vi "csmdoc_import_all_csm_VI_description_doc.vi"() -> ()   [LabVIEW 2017, in "csmdoc.lvlib"]
uses:
  csmdoc.lvlib
  _Shared/CSM Shared.lvlib
panel:
  out "Numeric":i32=317
  in  "LANG ID":string="EN"
  in  "Error in":errorcluster caption="error in (no error)"
  out "error out":errorcluster
  out "Array":path[](array[path])
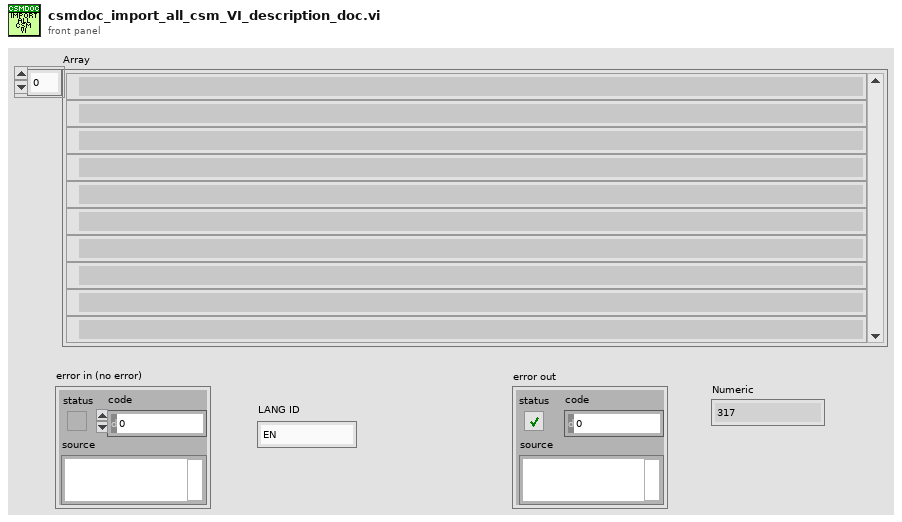
[diagram p1: front panel]
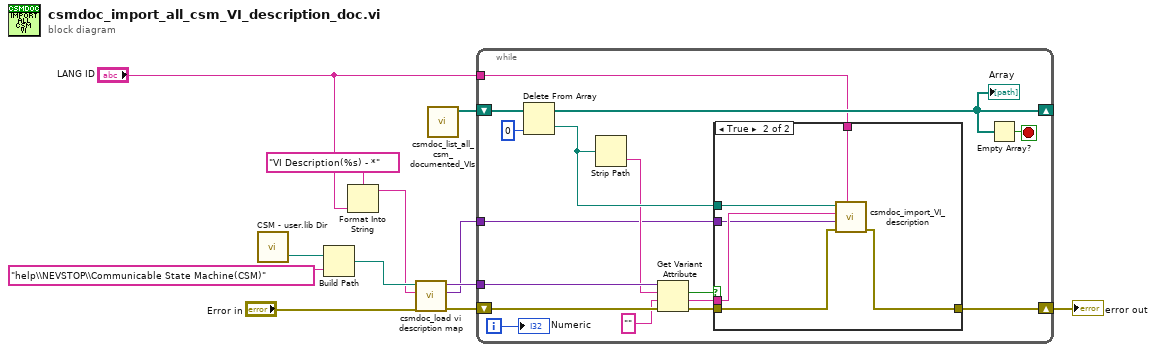
[diagram p0: block diagram]
diagram:
  n1 = call "CSM - user.lib Dir.vi"() -> ("<LabVIEW>"=w5:path)  [unwired: 2 in, 1 out]
  n2 = Build Path(base path=w5, name or relative path="help\\NEVSTOP\\Communicable State Machine(CSM)") -> (appended path=w4:path)
  n3 = Format Into String(format string="VI Description(%s) - *" ("pattern"), "LANG ID") -> (resulting string=w1:string)  [unwired: 2 in, 1 out]
  n4 = call "csmdoc_load vi description map.vi"("Error In"="Error in", "Pattern"=w1, "Path"=w4) -> ("error out"=w10:errorcluster, "NoteMap"=w7:variant, "DescMap"=w11:variant)  [unwired: 6 in]
  n5 = call "csmdoc_list_all_csm_documented_VIs.vi"() -> ("Array"=w12:path[])  [unwired: 11 in]
  n6 = while {
    shift-right: [w25] -> _
    shift-left: w12 -> [w27]
    tunnel: w11 -> [w23]
    shift-right: [w18] -> w9
    shift-left: w10 -> [w20]
    tunnel: w7 -> [w15]
    tunnel: "LANG ID" -> [w14]
    i -> [w13]
    stop <- w26 stop-if-true
    n7 = Delete From Array(array=w27, index=0) -> (deleted portion=w28:path, array with subset deleted=w25:path[])  [unwired: 1 in]
    "Array" <- w25
    n8 = Strip Path(path=w28) -> (name=w22:string)  [unwired: 1 out]
    n9 = Get Variant Attribute(Variant=w23, name=w22, default value (empty Variant)="" ("String"), error in=w20) -> (found=w21:bool, value=w16:string, error out=w19:errorcluster)  [unwired: 1 out]
    n10 = case shown="True" w21 {
      tunnel: w28 -> [_ w35]
      tunnel: w19 -> [w29 w34]
      tunnel: [w29 w33] -> w18
      tunnel: w16 -> [_ w32]
      tunnel: w15 -> [_ w31]
      tunnel: w14 -> [_ w30]
      frame False {
      }
      frame True {
        n11 = call "csmdoc_import_VI_description.vi"("LANG ID"=w30, "error in (no error)"=w34, "NOTE-Map"=w31, "String"=w32, "Path"=w35) -> ("error out"=w33:errorcluster)  [unwired: 6 in]
      }
    }
    n12 = Empty Array?(array=w25) -> (empty?=w26:bool)
    "Numeric" <- w13
  }
  "error out" <- w9
